vi "Set Disabled.vi"(8 "error in (no error)":errorcluster, 10 "Disabled":bool, 11 "NumericRangeBooleanIndicator in":refnum<class "NumericRangeBooleanIndicator.lvclass">) -> (0 "error out":errorcluster, 3 "NumericRangeBooleanIndicator out":refnum<class "NumericRangeBooleanIndicator.lvclass">)   [LabVIEW 2020, in "VolatusGUIElements.lvlib" / "NumericRangeBooleanIndicator.lvclass"]
uses:
  NumericRangeBooleanIndicator.lvclass
  NumericRangeBooleanIndicator.lvclass/NumericRangeBooleanIndicator.ctl
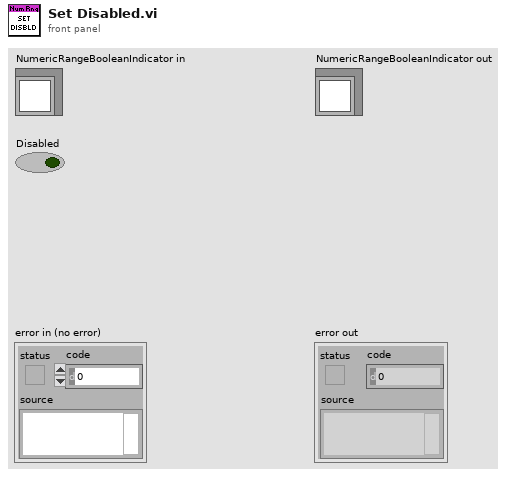
[diagram p1: front panel]
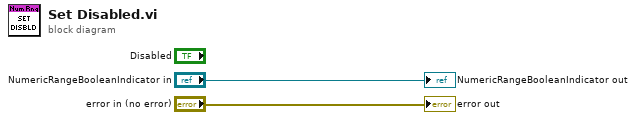
[diagram p0: block diagram]
diagram:
  "error out" <- "error in (no error)"
  "NumericRangeBooleanIndicator out" <- "NumericRangeBooleanIndicator in"
